vi "LabVIEW-Python-Interface_Example.vi"() -> ()   [LabVIEW 2016]
uses:
  pylvi/Controls/ArgumentType.ctl
  pylvi/Controls/DataType.ctl
  pylvi/Controls/ArgumentStructure.ctl
  pylvi/Controls/DescriptorStructure.ctl
  pylvi/PyLVi.lvclass
  <vilib>/Analysis/baseanly.llb/Mean (DBL).vi
  pylvi/argument_add/addArgument_Bool.vi
  pylvi/return_get/getReturn_Bool.vi
  pylvi/argument_add/addArgument_String.vi
  pylvi/return_get/getReturn_String.vi
  pylvi/argument_add/addArgument_Number_Float64.vi
  pylvi/return_get/getReturn_Number_Float64.vi
  pylvi/argument_add/addArgument_Number_Int32.vi
  pylvi/return_get/getReturn_Number_Int32.vi
  pylvi/argument_add/addArgument_Number_Complex128.vi
  pylvi/return_get/getReturn_Number_Complex128.vi
  pylvi/argument_add/addArgument_NumpyArray_Int32.vi
  pylvi/return_get/getReturn_NumpyArray_Int32.vi
  pylvi/argument_add/addArgument_NumpyArray_Float64.vi
  pylvi/return_get/getReturn_NumpyArray_Float64.vi
  pylvi/argument_add/addArgument_NumpyArray_Complex128.vi
  pylvi/return_get/getReturn_NumpyArray_Complex128.vi
  pylvi/argument_add/addArgument_NumpyArray2d_Int32.vi
  pylvi/return_get/getReturn_NumpyArray2d_Int32.vi
  pylvi/argument_add/addArgument_NumpyArray2d_Float64.vi
  pylvi/return_get/getReturn_NumpyArray2d_Float64.vi
  pylvi/argument_add/addArgument_NumpyArray2d_Complex128.vi
  pylvi/return_get/getReturn_NumpyArray2d_Complex128.vi
  pylvi/argument_add/addArgument_Dict.vi
  pylvi/return_get/getReturn_Dict.vi
  pylvi/attribute_set/setAttribute_Bool.vi
  pylvi/attribute_set/setAttribute_String.vi
  pylvi/attribute_set/setAttribute_Number_Int32.vi
  pylvi/attribute_set/setAttribute_Number_Float64.vi
  pylvi/attribute_set/setAttribute_Number_Complex128.vi
  pylvi/attribute_set/setAttribute_NumpyArray_Int32.vi
  pylvi/attribute_set/setAttribute_NumpyArray_Float64.vi
  pylvi/attribute_set/setAttribute_NumpyArray_Complex128.vi
  pylvi/attribute_set/setAttribute_NumpyArray2d_Int32.vi
  pylvi/attribute_set/setAttribute_NumpyArray2d_Float64.vi
  pylvi/attribute_set/setAttribute_NumpyArray2d_Complex128.vi
  pylvi/attribute_set/setAttribute_Dict.vi
  pylvi/attribute_get/getAttribute_Bool.vi
  pylvi/attribute_get/getAttribute_String.vi
  pylvi/attribute_get/getAttribute_Number_Int32.vi
  pylvi/attribute_get/getAttribute_Number_Float64.vi
  pylvi/attribute_get/getAttribute_Number_Complex128.vi
  pylvi/attribute_get/getAttribute_NumpyArray_Int32.vi
  pylvi/attribute_get/getAttribute_NumpyArray_Float64.vi
  pylvi/attribute_get/getAttribute_NumpyArray_Complex128.vi
  pylvi/attribute_get/getAttribute_NumpyArray2d_Int32.vi
  pylvi/attribute_get/getAttribute_NumpyArray2d_Float64.vi
  pylvi/attribute_get/getAttribute_NumpyArray2d_Complex128.vi
  pylvi/attribute_get/getAttribute_Dict.vi
  <vilib>/Analysis/NI_AALBase.lvlib
panel:
  in  "Tab Control":T1(tab)=enum."Single Argument Function Call"
  in  "open connection":bool
  in  "TCP address":string="tcp://127.0.0.1:5555"
  out "connection status":bool=TRUE
  in  "close connection":bool
  out "single:2darray receive complex":cdb[][](array[numeric])=[[2.0+0.0i, 2.0+0.0i, 4.0+0.0i, 4.0+0.0i]] caption="2darray receive complex"
  in  "single:2darray send complex":cdb[][](array[numeric])=[[2.17+0.25i, 2.0+0.0i, 4.0+0.88i, 4.0+0.0i], [0.5+0.0i, 85.6+0.0i, 7.2+1.52i, 0.0+0.0i]] caption="2darray send complex"
  out "single:array receive complex":cdb[](array[numeric]) caption="array receive complex"
  in  "single:array send complex":cdb[](array[numeric])=array[100005 elements] caption="array send complex"
  out "single:numeric receive complex":cdb caption="numeric receive complex"
  in  "single:numeric send complex":cdb=14.2+0.25i caption="numeric send complex"
  out "single:2darray receive":dbl[][](array[numeric])=[[2.0, 2.0, 4.0, 4.0]] caption="2darray receive"
  in  "single:2darray send":dbl[][](array[numeric])=[[0.85, 2.0, 4.0, 4.0], [0.0, 98.6, 9.58, 0.0]] caption="2darray send"
  in  "single:dict send":T2={"Name"="tcp://127.0.0.1:5555", "Number"=0.0, "Boolean"=FALSE, "Array"=[2.9, 2.0, 85.7, 4.01]} caption="dict send"
  out "single:dict receive":T2={"Name"="tcp://127.0.0.1:5555", "Number"=0.0, "Boolean"=FALSE, "Array"=[2.0, 2.0, 4.0, 4.0]} caption="dict receive"
  in  "single:function":string="fct_boolean" caption="function"
  in  "single:object":string="test" caption="object"
  in  "single:interations":i32=10 caption="interations"
  out "single:current iteration":i32=9 caption="current iteration"
  out "single:avg runtime [ms]":dbl=52.0 caption="avg runtime [ms]" format="%0.2f"
  in  "single argument fct call":bool
  in  "single:argtype":T3 caption="argtype"
  in  "single:data type":T4 caption="data type"
  in  "single:array send":dbl[](array[numeric])=[2.0, 2.99, 4.0, 4.869] caption="array send"
  out "single:array receive":dbl[](array[numeric]) caption="array receive"
  in  "single:bool send":bool caption="bool send"
  out "single:bool receive":bool caption="bool receive"
  in  "single:numeric send":dbl caption="numeric send"
  out "single:numeric receive":dbl caption="numeric receive"
  in  "single:string send":string caption="string send"
  out "single:string receive":string caption="string receive"
  out "multi:2darray receive complex":cdb[][](array[numeric])=[[4.0+170.6i, 4.0+0.2i, 8.0+1.6i, 8.0+0.0i], [0.0+0.0i, 3.0+104.0i, 0.0+1.1i, 0.0+0.0i]] caption="2darray receive complex"
  in  "multi:2darray send complex":cdb[][](array[numeric])=[[2.0+85.3i, 2.0+0.1i, 4.0+0.8i, 4.0+0.0i], [0.0+0.0i, 1.5+52.0i, 0.0+0.55i, 0.0+0.0i]] caption="2darray send complex"
  out "multi:array receive complex":cdb[](array[numeric])=[4.34+0.0i, 4.0+0.0i, 8.0+1.16i, 8.6+0.2i] caption="array receive complex"
  in  "multi:array send complex":cdb[](array[numeric])=[2.17+0.0i, 2.0+0.0i, 4.0+0.58i, 4.3+0.1i] caption="array send complex"
  out "multi:numeric receive complex":cdb=0.4+11.6i caption="numeric receive complex"
  in  "multi:numeric send complex":cdb=0.2+5.8i caption="numeric send complex"
  in  "multi:clear last argument":bool
  out "multi:argument receive":T5[](array[typedef])
  out "multi:2darray receive":dbl[][](array[numeric]) caption="2darray receive"
  out "multi:dict receive":T2={"Name"="tcp://127.0.0.1:5555", "Number"=0.0, "Boolean"=FALSE, "Array"=[2.0, 2.0, 4.0, 4.0]} caption="dict receive"
  out "multi:array receive":dbl[](array[numeric]) caption="array receive"
  out "multi:bool receive":bool caption="bool receive"
  out "multi:numeric receive":dbl caption="numeric receive"
  out "multi:string receive":string caption="string receive"
  in  "multi:get return parameter":bool
  in  "multi:add argument":bool
  in  "multi:call function":bool
  in  "multi:2darray send":dbl[][](array[numeric])=[[2.17, 2.0, 4.9, 4.0], [0.0, 8.5, 0.0, 0.0]] caption="2darray send"
  in  "multi:dict send":T2={"Name"="tcp://127.0.0.1:5555", "Number"=0.0, "Boolean"=FALSE, "Array"=[2.0, 2.0, 4.0, 4.0]} caption="dict send"
  in  "multi:array send":dbl[](array[numeric])=[28.5, 2.0, 85.3, 4.0] caption="array send"
  in  "multi:bool send":bool caption="bool send"
  in  "multi:numeric send":dbl caption="numeric send"
  in  "multi:string send":string caption="string send"
  in  "multi:function":string="multi_array_test" caption="function"
  in  "multi:object":string="test" caption="object"
  in  "multi:argtype":T3 caption="argtype"
  in  "multi:data type":T4 caption="data type"
  out "multi:argument send":T5[](array[typedef])
  out "prop:2darray receive complex":cdb[][](array[numeric])=[[2.0+0.0i, 2.0+0.0i, 4.0+0.0i, 4.0+0.0i], [0.0+0.0i, 0.0+0.0i, 1.2+0.22i, 0.0+0.0i]] caption="2darray get complex"
  in  "prop:2darray set complex":cdb[][](array[numeric])=[[2.0+0.25i, 2.68+17.2i, 4.0+0.98i, 4.0+0.0i], [8.6+52.8i, 0.0+0.0i, 1.2+0.22i, 0.0+0.0i]] caption="2darray set complex"
  out "prop:array get complex":cdb[](array[numeric])=[2.1+0.0i, 2.0+0.1i, 4.0+0.2i, 4.0+17.2i] caption="array get complex"
  in  "prop:array set complex":cdb[](array[numeric])=[2.1+0.0i, 2.0+0.1i, 4.0+0.2i, 4.0+17.2i] caption="array set complex"
  out "prop:numeric get complex":cdb=7.2+17.23i caption="numeric get complex"
  in  "prop:numeric set complex":cdb=25.5+0.72i caption="numeric set complex"
  out "prop:2darray get":dbl[][](array[numeric])=[[2.0, 2.0, 4.0, 4.0]] caption="2darray get"
  out "prop:dict get":T2={"Name"="tcp://127.0.0.1:5555", "Number"=0.0, "Boolean"=FALSE, "Array"=[2.0, 2.0, 4.0, 4.0]} caption="dict get"
  out "prop:array get":dbl[](array[numeric]) caption="array get"
  out "prop:bool get":bool caption="bool get"
  out "prop:numeric get":dbl caption="numeric get"
  out "grop:string get":string caption="string get"
  in  "prop:get":bool
  in  "prop:set":bool
  in  "prop:2darray set":dbl[][](array[numeric])=[[2.17, 2.9, 4.0, 4.0], [0.33, 0.0, 17.5, 0.0]] caption="2darray set"
  in  "prop:array set":dbl[](array[numeric])=[2.0, 2.0, 4.0, 4.0] caption="array set"
  in  "prop:dict set":T2={"Name"="tcp://127.0.0.1:5555", "Number"=0.0, "Boolean"=FALSE, "Array"=[2.5, 18.5, 8.5, 4.0]} caption="dict set"
  in  "prop:bool set":bool caption="bool set"
  in  "prop:numeric set":dbl caption="numeric set"
  in  "prop:string set":string caption="string set"
  in  "prop:property":string="var_double" caption="property/attribute"
  in  "prop:object":string="test" caption="object"
  in  "prop:argtype":T3=enum."numeric" caption="argtype"
  in  "prop:data type":T4=enum."float64" caption="data type"
  in  "stop":bool
  # "A function with a single parameter is called. This function returns the same value or a modified one."
  # "Benchmarking"
  # "1. Add arguments\n2. Call function\n3. Parse return parameters"
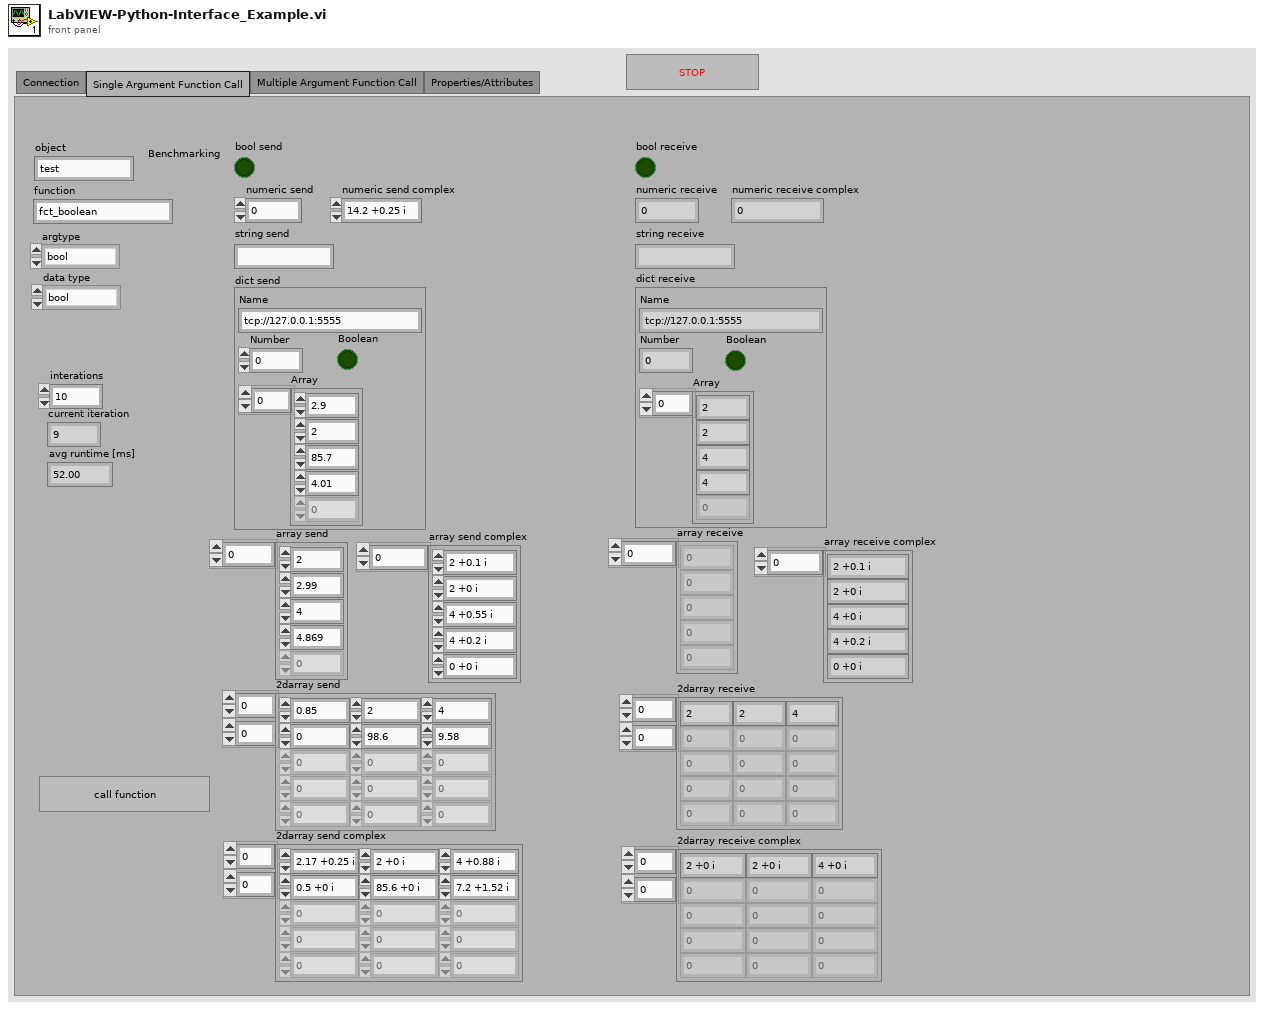
[diagram p1: front panel]
types:
  T1 = enum32{"Connection", "Single Argument Function Call", "Multiple Argument Function Call", "Properties/Attributes"}
  T2 = cluster{"Name":string, "Number":dbl, "Boolean":bool, "Array":dbl[]}
  T3 = typedef "PyLVi.lvlib/PyLVi.lvclass/ArgumentType.ctl" = enum8{"bool", "numeric", "string", "dict", "ndarray", "ndarray2d"}
  T4 = typedef "PyLVi.lvlib/PyLVi.lvclass/DataType.ctl" = enum16{"bool", "string", "int16", "int32", "float32", "float64", "complex128"}
  T5 = typedef "PyLVi.lvlib/PyLVi.lvclass/ArgumentStructure.ctl" = cluster{"descriptor structure":T6, "data string":string}
  T6 = typedef "PyLVi.lvlib/PyLVi.lvclass/DescriptorStructure.ctl" = cluster{"argtype":string, "dtype":string, "shape":u32[], "argname":string}
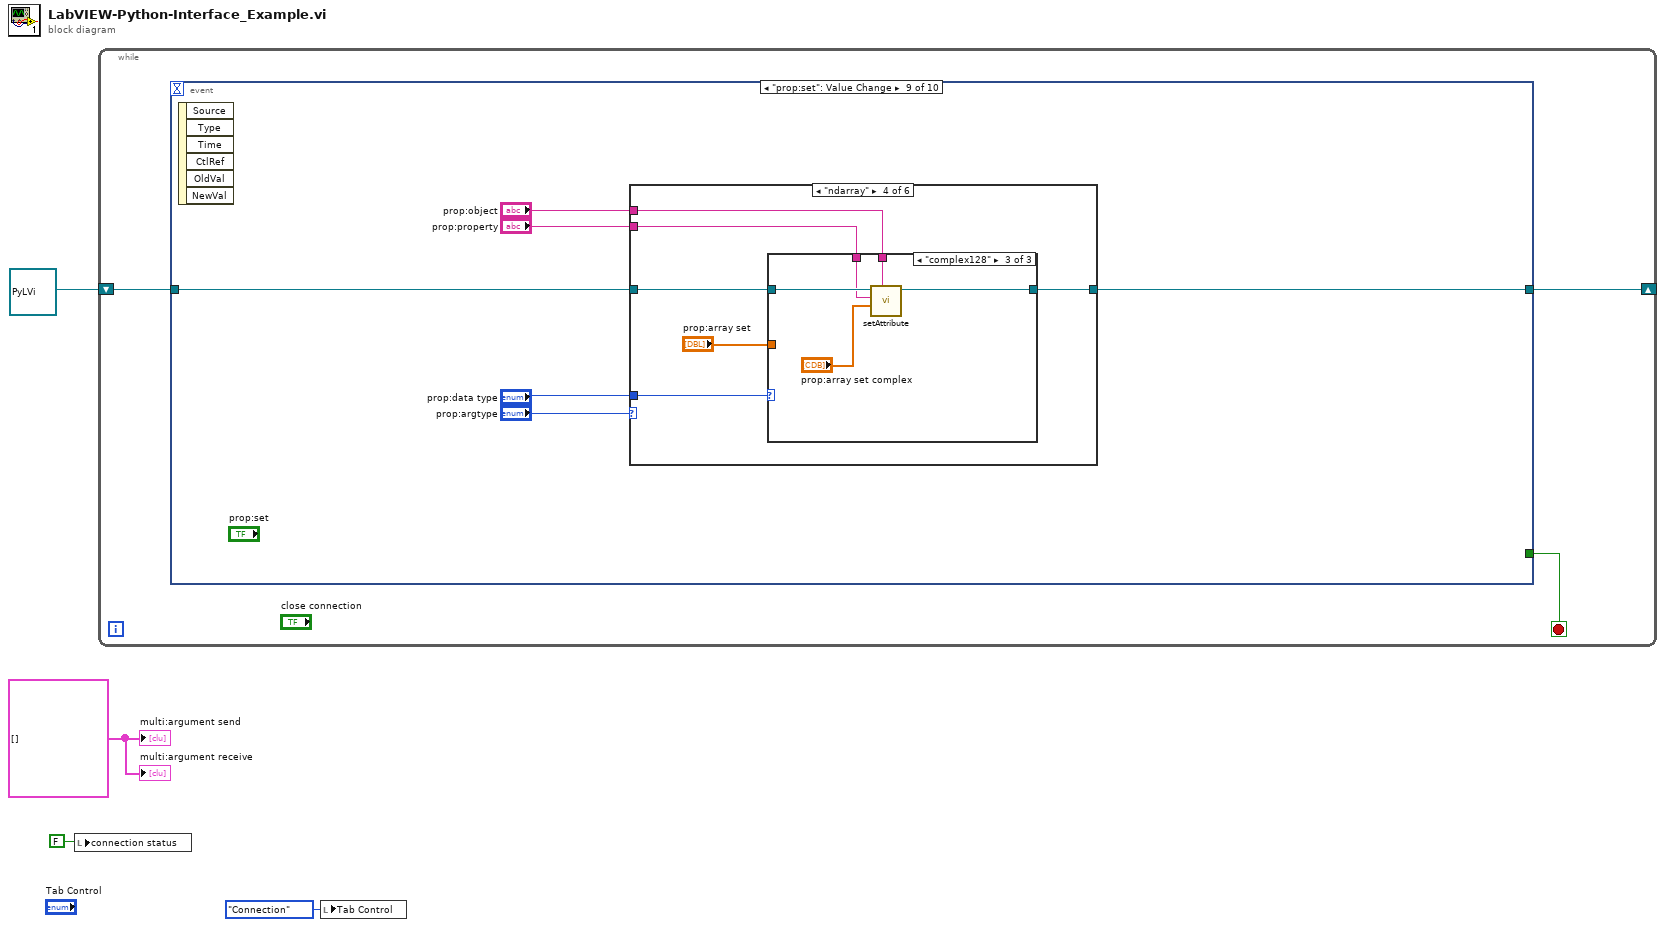
[diagram p0: block diagram]
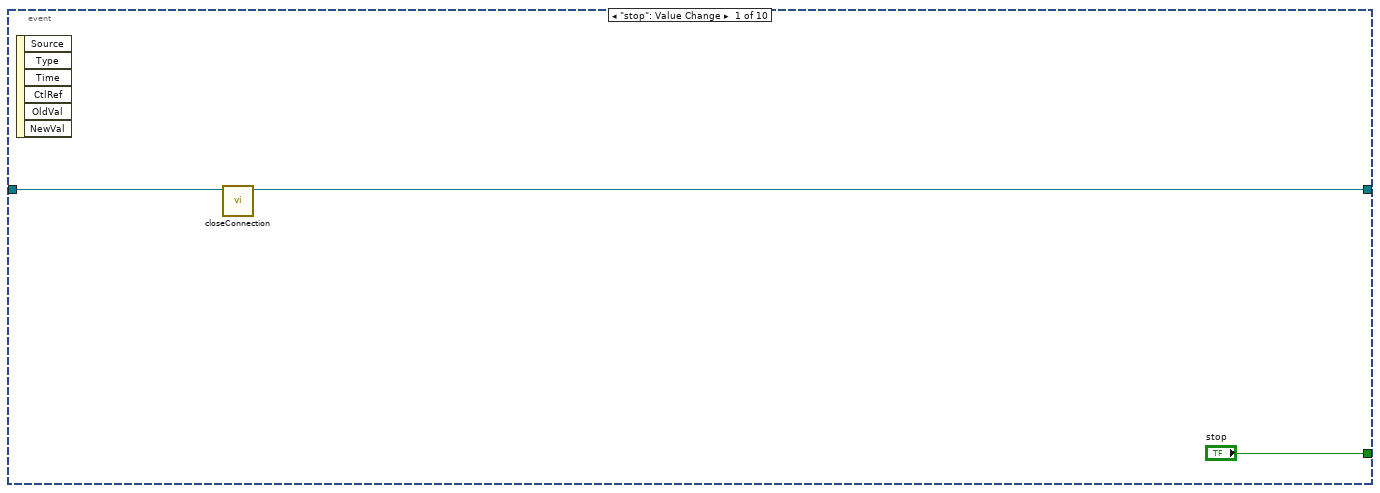
[diagram p2: hidden frame]
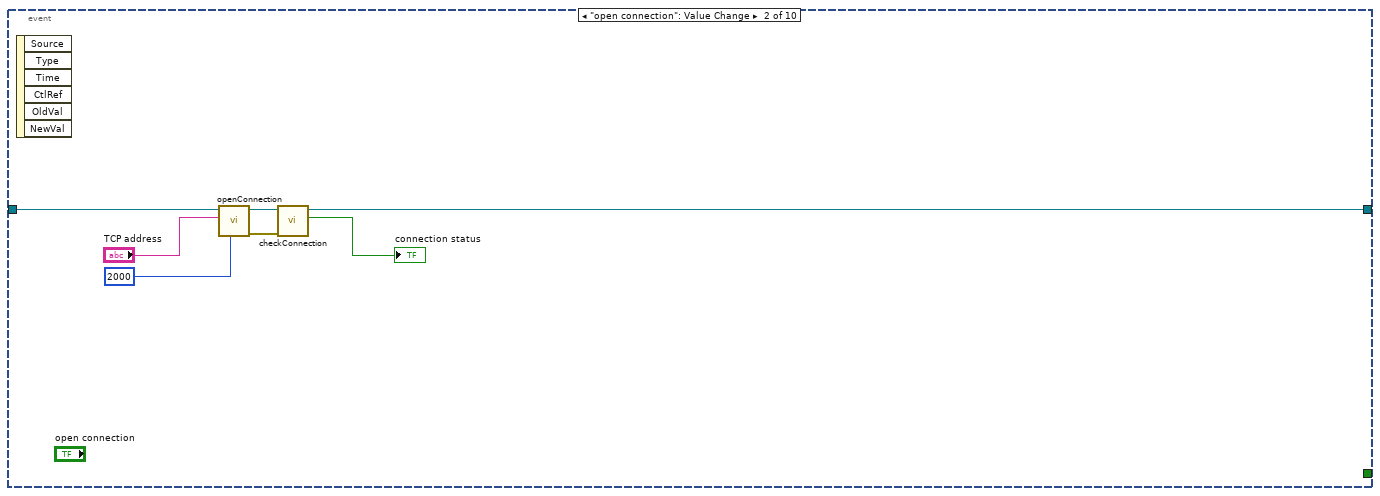
[diagram p3: hidden frame]
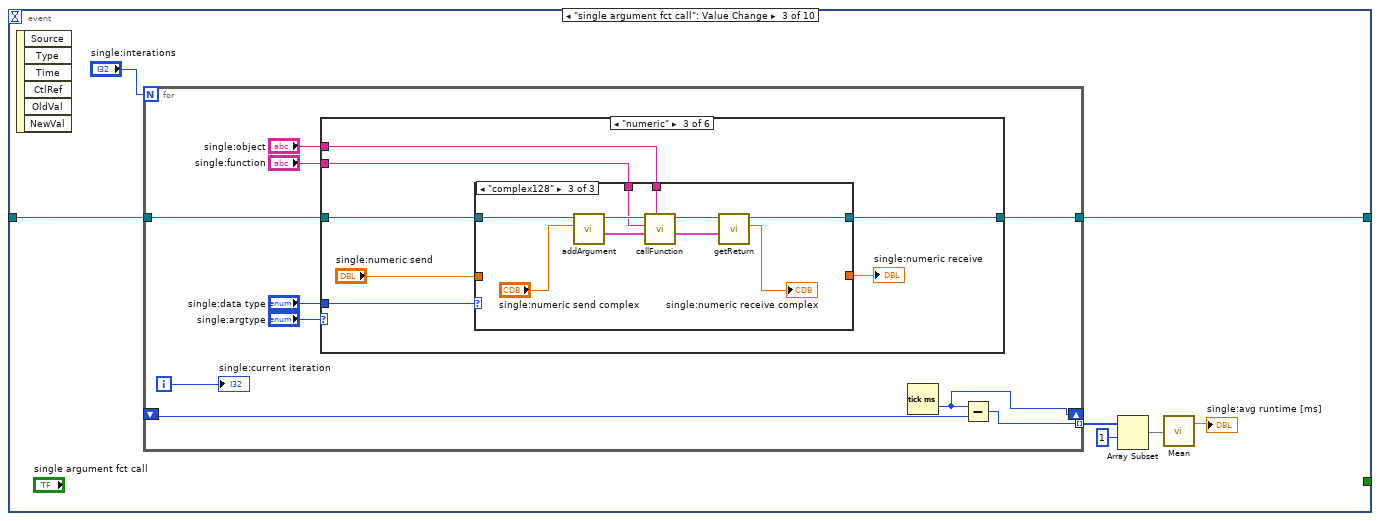
[diagram p4: hidden frame]
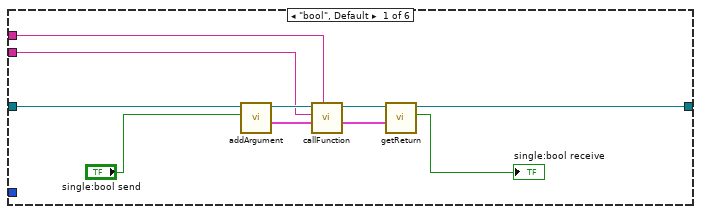
[diagram p5: hidden frame]
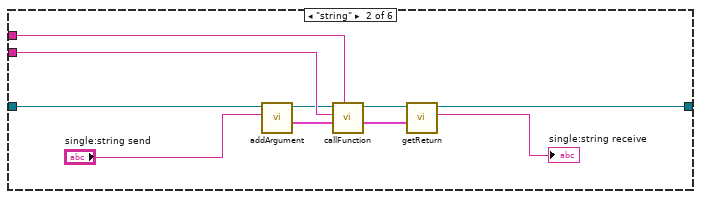
[diagram p6: hidden frame]
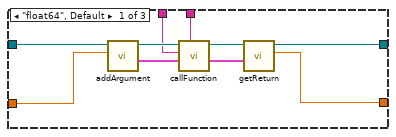
[diagram p7: hidden frame]
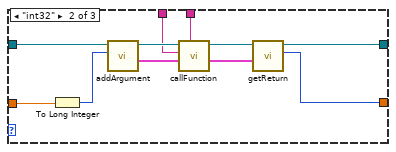
[diagram p8: hidden frame]
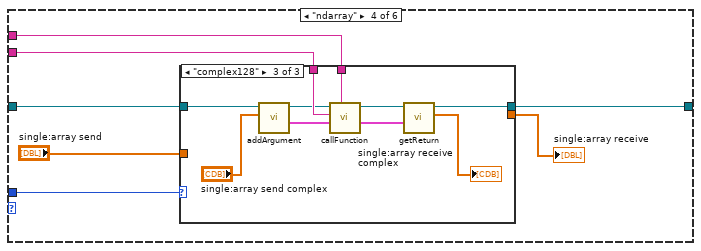
[diagram p9: hidden frame]
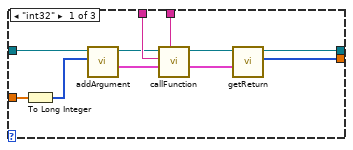
[diagram p10: hidden frame]
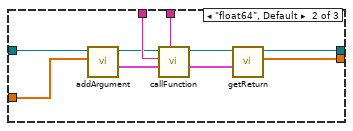
[diagram p11: hidden frame]
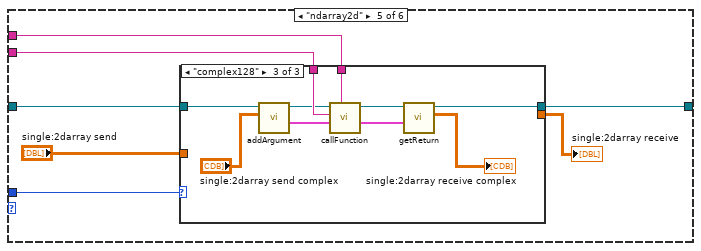
[diagram p12: hidden frame]
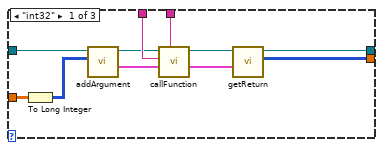
[diagram p13: hidden frame]
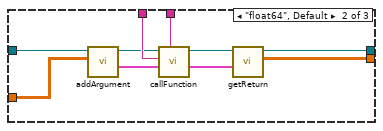
[diagram p14: hidden frame]
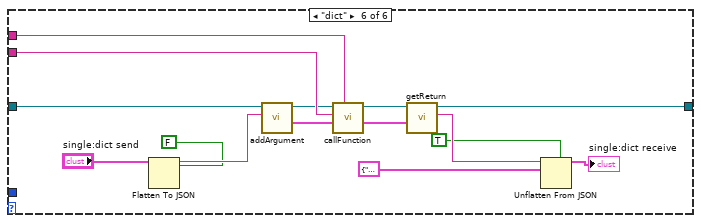
[diagram p15: hidden frame]
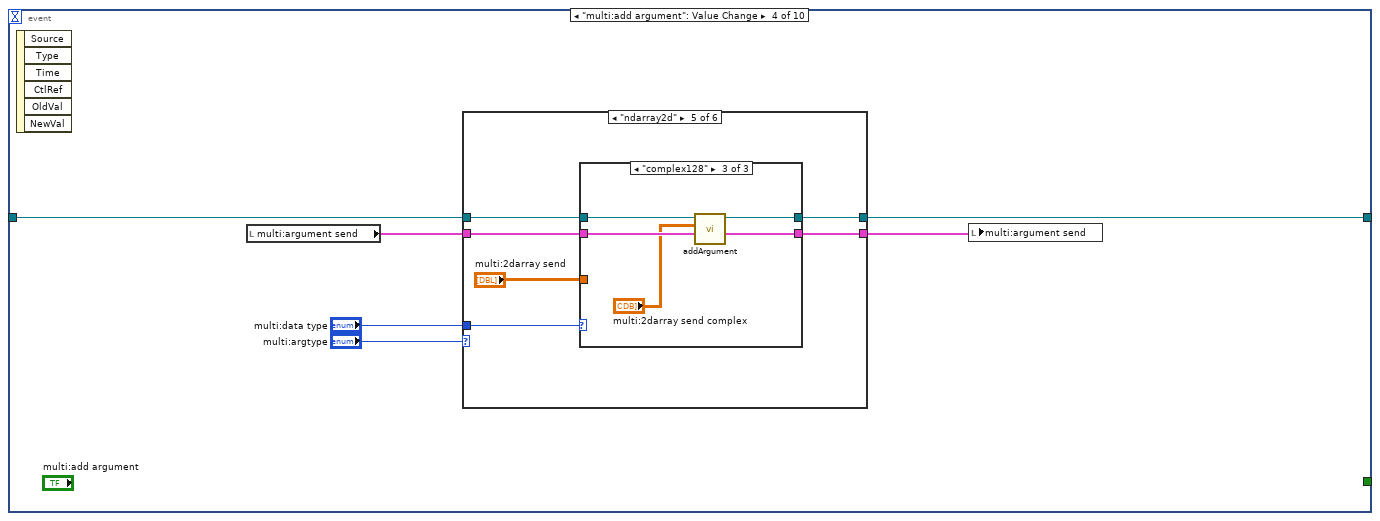
[diagram p16: hidden frame]
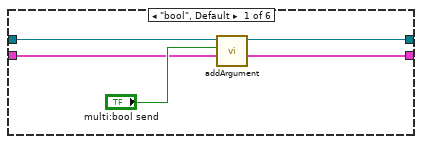
[diagram p17: hidden frame]
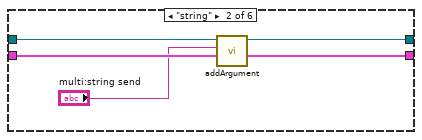
[diagram p18: hidden frame]
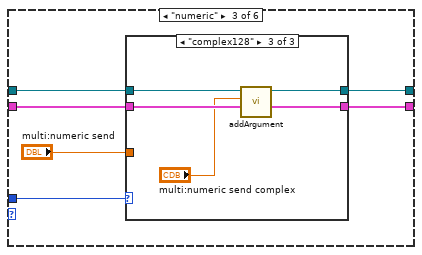
[diagram p19: hidden frame]
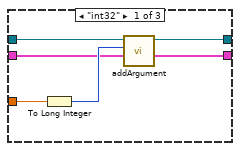
[diagram p20: hidden frame]
diagram:
  w2 = T5[] [] ("multi:argument send")
  n1 = local write "connection status"(FALSE ("status")) -> ()
  n2 = while {
    shift-right: [w6] -> _
    shift-left: refnum<class "PyLVi.lvclass"> refnum ("Python_LabView_Interface:Python-Labview_Communication.lvclass") -> [w5]
    stop <- w7 stop-if-true
    n3 = event shown="[8] \"prop:set\": Value Change" {
      selector: _ -> [_ _ _ _ _ _ _ _ _ _]
      dyn-events: _ -> [_ _ _ _ _ _ _ _ _ _]
      timeout: _ -> [_ _ _ _ _ _ _ _ _ _]
      tunnel: ["stop" _ _ _ _ _ _ _ _ _] -> w7
      tunnel: w5 -> [w9 w17 w24 w189 w273 w284 w290 w373 w378 w468]
      tunnel: [w8 w12 w23 w188 w273 w283 w289 w372 w374 w467] -> w6
      event "stop": Value Change {
        n4 = event-data() -> ()  [unwired: 1 in, 6 out]
        n5 = call "closeConnection.vi"("LabVIEW-Python-Interface in"=w9) -> ("LabVIEW-Python-Interface out"=w8:refnum<class "PyLVi.lvclass">)  [unwired: 9 in, 1 out]
      }
      event "open connection": Value Change {
        n6 = event-data() -> ()  [unwired: 1 in, 6 out]
        n7 = call "openConnection.vi"("recveive timeout"=2000, "TCP address"="TCP address", "LabVIEW-Python-Interface in"=w17) -> ("error out"=w14:errorcluster, "LabVIEW-Python-Interface out"=w15:refnum<class "PyLVi.lvclass">)  [unwired: 6 in, 1 out]
        n8 = call "checkConnection.vi"("error in (no error)"=w14, "LabVIEW-Python-Interface in"=w15) -> ("connection established"=→"connection status":bool, "LabVIEW-Python-Interface out"=w12:refnum<class "PyLVi.lvclass">)  [unwired: 7 in, 1 out]
      }
      event "single argument fct call": Value Change {
        n9 = event-data() -> ()  [unwired: 1 in, 6 out]
        n10 = for {
          N: "single:interations" -> [_]
          tunnel: w24 -> [w30]
          tunnel: [w31] -> w23
          shift-right: [w33] -> _
          shift-left: _ -> [w34]
          tunnel: [w32] -> w20 mode=indexing
          i -> [w25]
          n11 = case shown="\"numeric\"" "single:argtype" {
            tunnel: [w39 w53 w60 w99 w137 w182] -> w31
            tunnel: w30 -> [w40 w54 w61 w98 w136 w183]
            tunnel: "single:object" -> [w38 w52 w59 w97 w135 w181]
            tunnel: "single:function" -> [w37 w51 w58 w96 w134 w180]
            tunnel: "single:data type" -> [_ _ w57 w95 w133 _]
            frame "bool", Default {
              n12 = call-poly "addArgument.vi"("data"="single:bool send", "LabVIEW-Python-Interface in"=w40) -> ("argument list out"=w43:T5[], "LabVIEW-Python-Interface out"=w44:refnum<class "PyLVi.lvclass">)  [unwired: 7 in, 1 out]
              n13 = call "callFunction.vi"("object"=w38, "argument list in"=w43, "function"=w37, "LabVIEW-Python-Interface in"=w44) -> ("return list"=w41:T5[], "LabVIEW-Python-Interface out"=w42:refnum<class "PyLVi.lvclass">)  [unwired: 5 in, 1 out]
              n14 = call-poly "getReturn.vi"("return list in"=w41, "LabVIEW-Python-Interface in"=w42) -> ("data"=→"single:bool receive":bool, "LabVIEW-Python-Interface out"=w39:refnum<class "PyLVi.lvclass">)  [unwired: 6 in, 2 out]
            }
            frame "string" {
              n15 = call-poly "addArgument.vi"("data"="single:string send", "LabVIEW-Python-Interface in"=w54) -> ("argument list out"=w49:T5[], "LabVIEW-Python-Interface out"=w50:refnum<class "PyLVi.lvclass">)  [unwired: 7 in, 1 out]
              n16 = call "callFunction.vi"("object"=w52, "argument list in"=w49, "function"=w51, "LabVIEW-Python-Interface in"=w50) -> ("return list"=w47:T5[], "LabVIEW-Python-Interface out"=w48:refnum<class "PyLVi.lvclass">)  [unwired: 5 in, 1 out]
              n17 = call-poly "getReturn.vi"("return list in"=w47, "LabVIEW-Python-Interface in"=w48) -> ("data out"=→"single:string receive":string, "LabVIEW-Python-Interface out"=w53:refnum<class "PyLVi.lvclass">)  [unwired: 6 in, 2 out]
            }
            frame "numeric" {
              n18 = case shown="\"complex128\"" w57 {
                tunnel: w61 -> [w67 w78 w88]
                tunnel: [w66 w77 w87] -> w60
                tunnel: w59 -> [w65 w76 w86]
                tunnel: w58 -> [w64 w75 w85]
                tunnel: "single:numeric send" -> [w62 w72 _]
                tunnel: [w63 w74 _] -> w55
                frame "float64", Default {
                  n19 = call-poly "addArgument.vi"("data"=w62, "LabVIEW-Python-Interface in"=w67) -> ("argument list out"=w70:T5[], "LabVIEW-Python-Interface out"=w71:refnum<class "PyLVi.lvclass">)  [unwired: 7 in, 1 out]
                  n20 = call "callFunction.vi"("object"=w65, "argument list in"=w70, "function"=w64, "LabVIEW-Python-Interface in"=w71) -> ("return list"=w68:T5[], "LabVIEW-Python-Interface out"=w69:refnum<class "PyLVi.lvclass">)  [unwired: 5 in, 1 out]
                  n21 = call-poly "getReturn.vi"("return list in"=w68, "LabVIEW-Python-Interface in"=w69) -> ("data out"=w63:dbl, "LabVIEW-Python-Interface out"=w66:refnum<class "PyLVi.lvclass">)  [unwired: 6 in, 2 out]
                }
                frame "int32" {
                  n22 = To Long Integer(number=w72) -> (32bit integer=w73:i32)
                  n23 = call-poly "addArgument.vi"("data"=w73, "LabVIEW-Python-Interface in"=w78) -> ("argument list out"=w81:T5[], "LabVIEW-Python-Interface out"=w82:refnum<class "PyLVi.lvclass">)  [unwired: 7 in, 1 out]
                  n24 = call "callFunction.vi"("object"=w76, "argument list in"=w81, "function"=w75, "LabVIEW-Python-Interface in"=w82) -> ("return list"=w79:T5[], "LabVIEW-Python-Interface out"=w80:refnum<class "PyLVi.lvclass">)  [unwired: 5 in, 1 out]
                  n25 = call-poly "getReturn.vi"("return list in"=w79, "LabVIEW-Python-Interface in"=w80) -> ("data out"=w74:i32, "LabVIEW-Python-Interface out"=w77:refnum<class "PyLVi.lvclass">)  [unwired: 6 in, 2 out]
                }
                frame "complex128" {
                  n26 = call-poly "addArgument.vi"("data"="single:numeric send complex", "LabVIEW-Python-Interface in"=w88) -> ("argument list out"=w91:T5[], "LabVIEW-Python-Interface out"=w92:refnum<class "PyLVi.lvclass">)  [unwired: 7 in, 1 out]
                  n27 = call "callFunction.vi"("object"=w86, "argument list in"=w91, "function"=w85, "LabVIEW-Python-Interface in"=w92) -> ("return list"=w89:T5[], "LabVIEW-Python-Interface out"=w90:refnum<class "PyLVi.lvclass">)  [unwired: 5 in, 1 out]
                  n28 = call-poly "getReturn.vi"("return list in"=w89, "LabVIEW-Python-Interface in"=w90) -> ("data out"=→"single:numeric receive complex":cdb, "LabVIEW-Python-Interface out"=w87:refnum<class "PyLVi.lvclass">)  [unwired: 6 in, 2 out]
                }
              }
              "single:numeric receive" <- w55
            }
            frame "ndarray" {
              n29 = case shown="\"complex128\"" w95 {
                tunnel: [w102 w114 w124] -> w99
                tunnel: w98 -> [w107 w118 w128]
                tunnel: w97 -> [w110 w120 w130]
                tunnel: w96 -> [w109 w119 w129]
                tunnel: "single:array send" -> [w108 w111 _]
                tunnel: [w100 w112 _] -> w93
                frame "int32" {
                  n30 = To Long Integer(number=w108) -> (32bit integer=w104:i32[])
                  n31 = call-poly "addArgument.vi"("data"=w104, "LabVIEW-Python-Interface in"=w107) -> ("argument list out"=w105:T5[], "LabVIEW-Python-Interface out"=w106:refnum<class "PyLVi.lvclass">)  [unwired: 7 in, 1 out]
                  n32 = call "callFunction.vi"("object"=w110, "argument list in"=w105, "function"=w109, "LabVIEW-Python-Interface in"=w106) -> ("return list"=w101:T5[], "LabVIEW-Python-Interface out"=w103:refnum<class "PyLVi.lvclass">)  [unwired: 5 in, 1 out]
                  n33 = call-poly "getReturn.vi"("return list in"=w101, "LabVIEW-Python-Interface in"=w103) -> ("data out"=w100:i32[], "LabVIEW-Python-Interface out"=w102:refnum<class "PyLVi.lvclass">)  [unwired: 6 in, 2 out]
                }
                frame "float64", Default {
                  n34 = call-poly "addArgument.vi"("data"=w111, "LabVIEW-Python-Interface in"=w118) -> ("argument list out"=w116:T5[], "LabVIEW-Python-Interface out"=w117:refnum<class "PyLVi.lvclass">)  [unwired: 7 in, 1 out]
                  n35 = call "callFunction.vi"("object"=w120, "argument list in"=w116, "function"=w119, "LabVIEW-Python-Interface in"=w117) -> ("return list"=w113:T5[], "LabVIEW-Python-Interface out"=w115:refnum<class "PyLVi.lvclass">)  [unwired: 5 in, 1 out]
                  n36 = call-poly "getReturn.vi"("return list in"=w113, "LabVIEW-Python-Interface in"=w115) -> ("data out"=w112:dbl[], "LabVIEW-Python-Interface out"=w114:refnum<class "PyLVi.lvclass">)  [unwired: 6 in, 2 out]
                }
                frame "complex128" {
                  n37 = call-poly "addArgument.vi"("data"="single:array send complex", "LabVIEW-Python-Interface in"=w128) -> ("argument list out"=w126:T5[], "LabVIEW-Python-Interface out"=w127:refnum<class "PyLVi.lvclass">)  [unwired: 7 in, 1 out]
                  n38 = call "callFunction.vi"("object"=w130, "argument list in"=w126, "function"=w129, "LabVIEW-Python-Interface in"=w127) -> ("return list"=w123:T5[], "LabVIEW-Python-Interface out"=w125:refnum<class "PyLVi.lvclass">)  [unwired: 5 in, 1 out]
                  n39 = call-poly "getReturn.vi"("return list in"=w123, "LabVIEW-Python-Interface in"=w125) -> ("data out"=→"single:array receive complex":cdb[], "LabVIEW-Python-Interface out"=w124:refnum<class "PyLVi.lvclass">)  [unwired: 6 in, 2 out]
                }
              }
              "single:array receive" <- w93
            }
            frame "ndarray2d" {
              n40 = case shown="\"complex128\"" w133 {
                tunnel: [w140 w152 w162] -> w137
                tunnel: w136 -> [w145 w156 w166]
                tunnel: w135 -> [w148 w158 w168]
                tunnel: w134 -> [w147 w157 w167]
                tunnel: "single:2darray send" -> [w146 w149 _]
                tunnel: [w138 w150 _] -> w131
                frame "int32" {
                  n41 = To Long Integer(number=w146) -> (32bit integer=w142:i32[][])
                  n42 = call-poly "addArgument.vi"("data"=w142, "LabVIEW-Python-Interface in"=w145) -> ("argument list out"=w143:T5[], "LabVIEW-Python-Interface out"=w144:refnum<class "PyLVi.lvclass">)  [unwired: 7 in, 1 out]
                  n43 = call "callFunction.vi"("object"=w148, "argument list in"=w143, "function"=w147, "LabVIEW-Python-Interface in"=w144) -> ("return list"=w139:T5[], "LabVIEW-Python-Interface out"=w141:refnum<class "PyLVi.lvclass">)  [unwired: 5 in, 1 out]
                  n44 = call-poly "getReturn.vi"("return list in"=w139, "LabVIEW-Python-Interface in"=w141) -> ("data out"=w138:i32[][], "LabVIEW-Python-Interface out"=w140:refnum<class "PyLVi.lvclass">)  [unwired: 6 in, 2 out]
                }
                frame "float64", Default {
                  n45 = call-poly "addArgument.vi"("data"=w149, "LabVIEW-Python-Interface in"=w156) -> ("argument list out"=w154:T5[], "LabVIEW-Python-Interface out"=w155:refnum<class "PyLVi.lvclass">)  [unwired: 7 in, 1 out]
                  n46 = call "callFunction.vi"("object"=w158, "argument list in"=w154, "function"=w157, "LabVIEW-Python-Interface in"=w155) -> ("return list"=w151:T5[], "LabVIEW-Python-Interface out"=w153:refnum<class "PyLVi.lvclass">)  [unwired: 5 in, 1 out]
                  n47 = call-poly "getReturn.vi"("return list in"=w151, "LabVIEW-Python-Interface in"=w153) -> ("data out"=w150:dbl[][], "LabVIEW-Python-Interface out"=w152:refnum<class "PyLVi.lvclass">)  [unwired: 6 in, 2 out]
                }
                frame "complex128" {
                  n48 = call-poly "addArgument.vi"("data"="single:2darray send complex", "LabVIEW-Python-Interface in"=w166) -> ("argument list out"=w164:T5[], "LabVIEW-Python-Interface out"=w165:refnum<class "PyLVi.lvclass">)  [unwired: 7 in, 1 out]
                  n49 = call "callFunction.vi"("object"=w168, "argument list in"=w164, "function"=w167, "LabVIEW-Python-Interface in"=w165) -> ("return list"=w161:T5[], "LabVIEW-Python-Interface out"=w163:refnum<class "PyLVi.lvclass">)  [unwired: 5 in, 1 out]
                  n50 = call-poly "getReturn.vi"("return list in"=w161, "LabVIEW-Python-Interface in"=w163) -> ("data out"=→"single:2darray receive complex":cdb[][], "LabVIEW-Python-Interface out"=w162:refnum<class "PyLVi.lvclass">)  [unwired: 6 in, 2 out]
                }
              }
              "single:2darray receive" <- w131
            }
            frame "dict" {
              n51 = Flatten To JSON(enable LabVIEW extensions? (T)=FALSE, anything="single:dict send") -> (JSON string=w174:string)  [unwired: 1 in, 1 out]
              n52 = call-poly "addArgument.vi"("JSON string"=w174, "LabVIEW-Python-Interface in"=w183) -> ("argument list out"=w178:T5[], "LabVIEW-Python-Interface out"=w179:refnum<class "PyLVi.lvclass">)  [unwired: 7 in, 1 out]
              n53 = call "callFunction.vi"("object"=w181, "argument list in"=w178, "function"=w180, "LabVIEW-Python-Interface in"=w179) -> ("return list"=w176:T5[], "LabVIEW-Python-Interface out"=w177:refnum<class "PyLVi.lvclass">)  [unwired: 5 in, 1 out]
              n54 = call-poly "getReturn.vi"("return list in"=w176, "LabVIEW-Python-Interface in"=w177) -> ("data out"=w175:string, "LabVIEW-Python-Interface out"=w182:refnum<class "PyLVi.lvclass">)  [unwired: 6 in, 2 out]
              n55 = Unflatten From JSON(enable LabVIEW extensions? (T)=TRUE, JSON string=w175, type and defaults=T2 {"Name"="tcp://127.0.0.1:5555", "Number"=0.0, "Boolean"=FALSE, "Array"=[2.0, 2.0, 4.0, 4.0]} ("single:dict receive")) -> (value=→"single:dict receive":T2)  [unwired: 4 in, 1 out]
            }
          }
          n56 = Tick Count (ms)() -> (millisecond timer value=w33:u32)
          n57 = Subtract(x=w33, y=w34) -> (x-y=w32:u32)
          "single:current iteration" <- w25
        }
        n58 = Array Subset(array=w20, index=1) -> (w21:u32[])  [unwired: 1 in]
        n59 = call-poly <vilib>:"Mean.vi"("X"=w21) -> ("mean"=→"single:avg runtime [ms]":dbl)  [unwired: 1 out]
      }
      event "multi:add argument": Value Change {
        n60 = event-data() -> ()  [unwired: 1 in, 6 out]
        n61 = local read "multi:argument send"() -> (w184:T5[])
        n62 = case shown="\"ndarray2d\"" "multi:argtype" {
          tunnel: w189 -> [w194 w199 w205 w227 w249 w272]
          tunnel: [w193 w198 w204 w226 w248 w271] -> w188
          tunnel: "multi:data type" -> [_ _ w203 w225 w247 _]
          tunnel: [w191 w197 w202 w224 w246 w270] -> w185
          tunnel: w184 -> [w190 w196 w200 w223 w245 w269]
          frame "bool", Default {
            n63 = call-poly "addArgument.vi"("argument list in"=w190, "data"="multi:bool send", "LabVIEW-Python-Interface in"=w194) -> ("argument list out"=w191:T5[], "LabVIEW-Python-Interface out"=w193:refnum<class "PyLVi.lvclass">)  [unwired: 6 in, 1 out]
          }
          frame "string" {
            n64 = call-poly "addArgument.vi"("argument list in"=w196, "data"="multi:string send", "LabVIEW-Python-Interface in"=w199) -> ("argument list out"=w197:T5[], "LabVIEW-Python-Interface out"=w198:refnum<class "PyLVi.lvclass">)  [unwired: 6 in, 1 out]
          }
          frame "numeric" {
            n65 = case shown="\"complex128\"" w203 {
              tunnel: w205 -> [w211 w216 w221]
              tunnel: [w210 w215 w220] -> w204
              tunnel: [w209 w214 w219] -> w202
              tunnel: "multi:numeric send" -> [w208 w213 _]
              tunnel: w200 -> [w206 w212 w218]
              frame "int32" {
                n66 = To Long Integer(number=w208) -> (32bit integer=w207:i32)
                n67 = call-poly "addArgument.vi"("argument list in"=w206, "data"=w207, "LabVIEW-Python-Interface in"=w211) -> ("argument list out"=w209:T5[], "LabVIEW-Python-Interface out"=w210:refnum<class "PyLVi.lvclass">)  [unwired: 6 in, 1 out]
              }
              frame "float64", Default {
                n68 = call-poly "addArgument.vi"("argument list in"=w212, "data"=w213, "LabVIEW-Python-Interface in"=w216) -> ("argument list out"=w214:T5[], "LabVIEW-Python-Interface out"=w215:refnum<class "PyLVi.lvclass">)  [unwired: 6 in, 1 out]
              }
              frame "complex128" {
                n69 = call-poly "addArgument.vi"("argument list in"=w218, "data"="multi:numeric send complex", "LabVIEW-Python-Interface in"=w221) -> ("argument list out"=w219:T5[], "LabVIEW-Python-Interface out"=w220:refnum<class "PyLVi.lvclass">)  [unwired: 6 in, 1 out]
              }
            }
          }
          frame "ndarray" {
            n70 = case shown="\"complex128\"" w225 {
              tunnel: w227 -> [w233 w238 w243]
              tunnel: [w232 w237 w242] -> w226
              tunnel: [w231 w236 w241] -> w224
              tunnel: "multi:array send" -> [w230 w235 _]
              tunnel: w223 -> [w228 w234 w240]
              frame "int32" {
                n71 = To Long Integer(number=w230) -> (32bit integer=w229:i32[])
                n72 = call-poly "addArgument.vi"("argument list in"=w228, "data"=w229, "LabVIEW-Python-Interface in"=w233) -> ("argument list out"=w231:T5[], "LabVIEW-Python-Interface out"=w232:refnum<class "PyLVi.lvclass">)  [unwired: 6 in, 1 out]
              }
              frame "float64", Default {
                n73 = call-poly "addArgument.vi"("argument list in"=w234, "data"=w235, "LabVIEW-Python-Interface in"=w238) -> ("argument list out"=w236:T5[], "LabVIEW-Python-Interface out"=w237:refnum<class "PyLVi.lvclass">)  [unwired: 6 in, 1 out]
              }
              frame "complex128" {
                n74 = call-poly "addArgument.vi"("argument list in"=w240, "data"="multi:array send complex", "LabVIEW-Python-Interface in"=w243) -> ("argument list out"=w241:T5[], "LabVIEW-Python-Interface out"=w242:refnum<class "PyLVi.lvclass">)  [unwired: 6 in, 1 out]
              }
            }
          }
          frame "ndarray2d" {
            n75 = case shown="\"complex128\"" w247 {
              tunnel: w249 -> [w255 w260 w265]
              tunnel: [w254 w259 w264] -> w248
              tunnel: [w253 w258 w263] -> w246
              tunnel: "multi:2darray send" -> [w252 w257 _]
              tunnel: w245 -> [w250 w256 w262]
              frame "int32" {
                n76 = To Long Integer(number=w252) -> (32bit integer=w251:i32[][])
                n77 = call-poly "addArgument.vi"("argument list in"=w250, "data"=w251, "LabVIEW-Python-Interface in"=w255) -> ("argument list out"=w253:T5[], "LabVIEW-Python-Interface out"=w254:refnum<class "PyLVi.lvclass">)  [unwired: 6 in, 1 out]
              }
              frame "float64", Default {
                n78 = call-poly "addArgument.vi"("argument list in"=w256, "data"=w257, "LabVIEW-Python-Interface in"=w260) -> ("argument list out"=w258:T5[], "LabVIEW-Python-Interface out"=w259:refnum<class "PyLVi.lvclass">)  [unwired: 6 in, 1 out]
              }
              frame "complex128" {
                n79 = call-poly "addArgument.vi"("argument list in"=w262, "data"="multi:2darray send complex", "LabVIEW-Python-Interface in"=w265) -> ("argument list out"=w263:T5[], "LabVIEW-Python-Interface out"=w264:refnum<class "PyLVi.lvclass">)  [unwired: 6 in, 1 out]
              }
            }
          }
          frame "dict" {
            n80 = Flatten To JSON(enable LabVIEW extensions? (T)=FALSE, anything="multi:dict send") -> (JSON string=w266:string)  [unwired: 1 in, 1 out]
            n81 = call-poly "addArgument.vi"("argument list in"=w269, "JSON string"=w266, "LabVIEW-Python-Interface in"=w272) -> ("argument list out"=w270:T5[], "LabVIEW-Python-Interface out"=w271:refnum<class "PyLVi.lvclass">)  [unwired: 6 in, 1 out]
          }
        }
        n82 = local write "multi:argument send"(w185) -> ()
      }
      event "multi:clear last argument": Value Change {
        # "delete last element"
        n83 = event-data() -> ()  [unwired: 1 in, 6 out]
        n84 = local read "multi:argument send"() -> (w276:T5[])
        n85 = Array Size(array=w276) -> (size(s)=w274:i32)
        n86 = Decrement(x=w274) -> (x-1=w275:i32)
        n87 = Delete From Array(array=w276, length=1, index=w275) -> (array with subset deleted=w278:T5[])  [unwired: 1 out]
        n88 = local write "multi:argument send"(w278) -> ()
      }
      event "multi:call function": Value Change {
        n89 = event-data() -> ()  [unwired: 1 in, 6 out]
        n90 = local read "multi:argument send"() -> (w280:T5[])
        n91 = call "callFunction.vi"("object"="multi:object", "argument list in"=w280, "function"="multi:function", "LabVIEW-Python-Interface in"=w284) -> ("return list"=w279:T5[], "LabVIEW-Python-Interface out"=w283:refnum<class "PyLVi.lvclass">)  [unwired: 5 in, 1 out]
        n92 = local write "multi:argument receive"(w279) -> ()
      }
      event "multi:get return parameter": Value Change {
        n93 = event-data() -> ()  [unwired: 1 in, 6 out]
        n94 = local read "multi:argument receive"() -> (w286:T5[])
        n95 = local read "multi:data type"() -> (w288:T4)
        n96 = local read "multi:argtype"() -> (w287:T3)
        n97 = case shown="\"ndarray2d\"" w287 {
          tunnel: w290 -> [w295 w300 w306 w327 w348 w371]
          tunnel: [w294 w299 w305 w326 w347 w370] -> w289
          tunnel: w288 -> [_ _ w304 w325 w346 _]
          tunnel: w286 -> [w293 w296 w303 w324 w345 w365]
          tunnel: [w292 w297 w302 w323 w344 w364] -> w285
          frame "bool", Default {
            n98 = call-poly "getReturn.vi"("return list in"=w293, "LabVIEW-Python-Interface in"=w295) -> ("return list out"=w292:T5[], "data"=→"multi:bool receive":bool, "LabVIEW-Python-Interface out"=w294:refnum<class "PyLVi.lvclass">)  [unwired: 6 in, 1 out]
          }
          frame "string" {
            n99 = call-poly "getReturn.vi"("return list in"=w296, "LabVIEW-Python-Interface in"=w300) -> ("return list out"=w297:T5[], "data out"=→"multi:string receive":string, "LabVIEW-Python-Interface out"=w299:refnum<class "PyLVi.lvclass">)  [unwired: 6 in, 1 out]
          }
          frame "numeric" {
            n100 = case shown="\"complex128\"" w304 {
              tunnel: w306 -> [w311 w316 w321]
              tunnel: [w310 w315 w320] -> w305
              tunnel: [w309 w314 _] -> w301
              tunnel: w303 -> [w308 w313 w319]
              tunnel: [w307 w312 w318] -> w302
              frame "int32" {
                n101 = call-poly "getReturn.vi"("return list in"=w308, "LabVIEW-Python-Interface in"=w311) -> ("return list out"=w307:T5[], "data out"=w309:i32, "LabVIEW-Python-Interface out"=w310:refnum<class "PyLVi.lvclass">)  [unwired: 6 in, 1 out]
              }
              frame "float64", Default {
                n102 = call-poly "getReturn.vi"("return list in"=w313, "LabVIEW-Python-Interface in"=w316) -> ("return list out"=w312:T5[], "data out"=w314:dbl, "LabVIEW-Python-Interface out"=w315:refnum<class "PyLVi.lvclass">)  [unwired: 6 in, 1 out]
              }
              frame "complex128" {
                n103 = call-poly "getReturn.vi"("return list in"=w319, "LabVIEW-Python-Interface in"=w321) -> ("return list out"=w318:T5[], "data out"=→"multi:numeric receive complex":cdb, "LabVIEW-Python-Interface out"=w320:refnum<class "PyLVi.lvclass">)  [unwired: 6 in, 1 out]
              }
            }
            "multi:numeric receive" <- w301
          }
          frame "ndarray" {
            n104 = case shown="\"complex128\"" w325 {
              tunnel: w327 -> [w332 w337 w342]
              tunnel: [w331 w336 w341] -> w326
              tunnel: [w330 w335 _] -> w322
              tunnel: w324 -> [w329 w334 w340]
              tunnel: [w328 w333 w339] -> w323
              frame "int32" {
                n105 = call-poly "getReturn.vi"("return list in"=w329, "LabVIEW-Python-Interface in"=w332) -> ("return list out"=w328:T5[], "data out"=w330:i32[], "LabVIEW-Python-Interface out"=w331:refnum<class "PyLVi.lvclass">)  [unwired: 6 in, 1 out]
              }
              frame "float64", Default {
                n106 = call-poly "getReturn.vi"("return list in"=w334, "LabVIEW-Python-Interface in"=w337) -> ("return list out"=w333:T5[], "data out"=w335:dbl[], "LabVIEW-Python-Interface out"=w336:refnum<class "PyLVi.lvclass">)  [unwired: 6 in, 1 out]
              }
              frame "complex128" {
                n107 = call-poly "getReturn.vi"("return list in"=w340, "LabVIEW-Python-Interface in"=w342) -> ("return list out"=w339:T5[], "data out"=→"multi:array receive complex":cdb[], "LabVIEW-Python-Interface out"=w341:refnum<class "PyLVi.lvclass">)  [unwired: 6 in, 1 out]
              }
            }
            "multi:array receive" <- w322
          }
          frame "ndarray2d" {
            n108 = case shown="\"complex128\"" w346 {
              tunnel: w348 -> [w353 w358 w363]
              tunnel: [w352 w357 w362] -> w347
              tunnel: [w351 w356 _] -> w343
              tunnel: w345 -> [w350 w355 w361]
              tunnel: [w349 w354 w360] -> w344
              frame "int32" {
                n109 = call-poly "getReturn.vi"("return list in"=w350, "LabVIEW-Python-Interface in"=w353) -> ("return list out"=w349:T5[], "data out"=w351:i32[][], "LabVIEW-Python-Interface out"=w352:refnum<class "PyLVi.lvclass">)  [unwired: 6 in, 1 out]
              }
              frame "float64", Default {
                n110 = call-poly "getReturn.vi"("return list in"=w355, "LabVIEW-Python-Interface in"=w358) -> ("return list out"=w354:T5[], "data out"=w356:dbl[][], "LabVIEW-Python-Interface out"=w357:refnum<class "PyLVi.lvclass">)  [unwired: 6 in, 1 out]
              }
              frame "complex128" {
                n111 = call-poly "getReturn.vi"("return list in"=w361, "LabVIEW-Python-Interface in"=w363) -> ("return list out"=w360:T5[], "data out"=→"multi:2darray receive complex":cdb[][], "LabVIEW-Python-Interface out"=w362:refnum<class "PyLVi.lvclass">)  [unwired: 6 in, 1 out]
              }
            }
            "multi:2darray receive" <- w343
          }
          frame "dict" {
            n112 = call-poly "getReturn.vi"("return list in"=w365, "LabVIEW-Python-Interface in"=w371) -> ("return list out"=w364:T5[], "data out"=w368:string, "LabVIEW-Python-Interface out"=w370:refnum<class "PyLVi.lvclass">)  [unwired: 6 in, 1 out]
            n113 = Unflatten From JSON(enable LabVIEW extensions? (T)=TRUE, JSON string=w368, type and defaults=T2 {"Name"="tcp://127.0.0.1:5555", "Number"=0.0, "Boolean"=FALSE, "Array"=[2.0, 2.0, 4.0, 4.0]} ("single:dict receive")) -> (value=→"multi:dict receive":T2)  [unwired: 4 in, 1 out]
          }
        }
        n114 = local write "multi:argument receive"(w285) -> ()
      }
      event "close connection": Value Change {
        n115 = event-data() -> ()  [unwired: 1 in, 6 out]
        n116 = call "closeConnection.vi"("LabVIEW-Python-Interface in"=w373) -> ("LabVIEW-Python-Interface out"=w372:refnum<class "PyLVi.lvclass">)  [unwired: 9 in, 1 out]
      }
      event "prop:set": Value Change {
        n117 = event-data() -> ()  [unwired: 1 in, 6 out]
        n118 = case shown="\"ndarray\"" "prop:argtype" {
          tunnel: w378 -> [w384 w389 w395 w417 w439 w462]
          tunnel: "prop:object" -> [w382 w387 w394 w416 w438 w460]
          tunnel: "prop:property" -> [w381 w386 w393 w415 w437 w459]
          tunnel: "prop:data type" -> [_ _ w392 w414 w436 _]
          tunnel: [w383 w388 w390 w413 w435 w461] -> w374
          frame "bool", Default {
            n119 = call-poly "setAttribute.vi"("object"=w382, "data"="prop:bool set", "attribute"=w381, "LabVIEW-Python-Interface in"=w384) -> ("LabVIEW-Python-Interface out"=w383:refnum<class "PyLVi.lvclass">)  [unwired: 6 in, 1 out]
          }
          frame "string" {
            n120 = call-poly "setAttribute.vi"("object"=w387, "data"="prop:string set", "attribute"=w386, "LabVIEW-Python-Interface in"=w389) -> ("LabVIEW-Python-Interface out"=w388:refnum<class "PyLVi.lvclass">)  [unwired: 6 in, 1 out]
          }
          frame "numeric" {
            n121 = case shown="\"complex128\"" w392 {
              tunnel: w395 -> [w401 w406 w411]
              tunnel: w394 -> [w400 w405 w410]
              tunnel: w393 -> [w399 w404 w409]
              tunnel: "prop:numeric set" -> [w396 w402 _]
              tunnel: [w397 w403 w408] -> w390
              frame "int32" {
                n122 = To Long Integer(number=w396) -> (32bit integer=w398:i32)
                n123 = call-poly "setAttribute.vi"("object"=w400, "data"=w398, "attribute"=w399, "LabVIEW-Python-Interface in"=w401) -> ("LabVIEW-Python-Interface out"=w397:refnum<class "PyLVi.lvclass">)  [unwired: 6 in, 1 out]
              }
              frame "float64", Default {
                n124 = call-poly "setAttribute.vi"("object"=w405, "data"=w402, "attribute"=w404, "LabVIEW-Python-Interface in"=w406) -> ("LabVIEW-Python-Interface out"=w403:refnum<class "PyLVi.lvclass">)  [unwired: 6 in, 1 out]
              }
              frame "complex128" {
                n125 = call-poly "setAttribute.vi"("object"=w410, "data"="prop:numeric set complex", "attribute"=w409, "LabVIEW-Python-Interface in"=w411) -> ("LabVIEW-Python-Interface out"=w408:refnum<class "PyLVi.lvclass">)  [unwired: 6 in, 1 out]
              }
            }
          }
          frame "ndarray" {
            n126 = case shown="\"complex128\"" w414 {
              tunnel: w417 -> [w423 w428 w433]
              tunnel: w416 -> [w422 w427 w432]
              tunnel: w415 -> [w421 w426 w431]
              tunnel: "prop:array set" -> [w419 w424 _]
              tunnel: [w418 w425 w430] -> w413
              frame "int32" {
                n127 = To Long Integer(number=w419) -> (32bit integer=w420:i32[])
                n128 = call-poly "setAttribute.vi"("object"=w422, "data"=w420, "attribute"=w421, "LabVIEW-Python-Interface in"=w423) -> ("LabVIEW-Python-Interface out"=w418:refnum<class "PyLVi.lvclass">)  [unwired: 6 in, 1 out]
              }
              frame "float64", Default {
                n129 = call-poly "setAttribute.vi"("object"=w427, "data"=w424, "attribute"=w426, "LabVIEW-Python-Interface in"=w428) -> ("LabVIEW-Python-Interface out"=w425:refnum<class "PyLVi.lvclass">)  [unwired: 6 in, 1 out]
              }
              frame "complex128" {
                n130 = call-poly "setAttribute.vi"("object"=w432, "data"="prop:array set complex", "attribute"=w431, "LabVIEW-Python-Interface in"=w433) -> ("LabVIEW-Python-Interface out"=w430:refnum<class "PyLVi.lvclass">)  [unwired: 6 in, 1 out]
              }
            }
          }
          frame "ndarray2d" {
            n131 = case shown="\"complex128\"" w436 {
              tunnel: w439 -> [w445 w450 w455]
              tunnel: w438 -> [w444 w449 w454]
              tunnel: w437 -> [w443 w448 w453]
              tunnel: "prop:2darray set" -> [w441 w446 _]
              tunnel: [w440 w447 w452] -> w435
              frame "int32" {
                n132 = To Long Integer(number=w441) -> (32bit integer=w442:i32[][])
                n133 = call-poly "setAttribute.vi"("object"=w444, "data"=w442, "attribute"=w443, "LabVIEW-Python-Interface in"=w445) -> ("LabVIEW-Python-Interface out"=w440:refnum<class "PyLVi.lvclass">)  [unwired: 6 in, 1 out]
              }
              frame "float64", Default {
                n134 = call-poly "setAttribute.vi"("object"=w449, "data"=w446, "attribute"=w448, "LabVIEW-Python-Interface in"=w450) -> ("LabVIEW-Python-Interface out"=w447:refnum<class "PyLVi.lvclass">)  [unwired: 6 in, 1 out]
              }
              frame "complex128" {
                n135 = call-poly "setAttribute.vi"("object"=w454, "data"="prop:2darray set complex", "attribute"=w453, "LabVIEW-Python-Interface in"=w455) -> ("LabVIEW-Python-Interface out"=w452:refnum<class "PyLVi.lvclass">)  [unwired: 6 in, 1 out]
              }
            }
          }
          frame "dict" {
            n136 = Flatten To JSON(enable LabVIEW extensions? (T)=FALSE, anything="prop:dict set") -> (JSON string=w457:string)  [unwired: 1 in, 1 out]
            n137 = call-poly "setAttribute.vi"("object"=w460, "data dict"=w457, "attribute"=w459, "LabVIEW-Python-Interface in"=w462) -> ("LabVIEW-Python-Interface out"=w461:refnum<class "PyLVi.lvclass">)  [unwired: 6 in, 1 out]
          }
        }
      }
      event "prop:get": Value Change {
        n138 = event-data() -> ()  [unwired: 1 in, 6 out]
        n139 = local read "prop:data type"() -> (w463:T4)
        n140 = local read "prop:property"() -> (w465:string)
        n141 = local read "prop:argtype"() -> (w464:T3)
        n142 = local read "prop:object"() -> (w466:string)
        n143 = case shown="\"numeric\"" w464 {
          tunnel: w468 -> [w473 w478 w484 w505 w526 w549]
          tunnel: [w472 w477 w483 w504 w525 w548] -> w467
          tunnel: w466 -> [w471 w476 w482 w503 w524 w547]
          tunnel: w465 -> [w470 w475 w481 w502 w523 w546]
          tunnel: w463 -> [_ _ w480 w501 w522 _]
          frame "bool", Default {
            n144 = call-poly "getAttribute.vi"("object"=w471, "attribute"=w470, "LabVIEW-Python-Interface in"=w473) -> ("data"=→"prop:bool get":bool, "LabVIEW-Python-Interface out"=w472:refnum<class "PyLVi.lvclass">)  [unwired: 6 in, 1 out]
          }
          frame "string" {
            n145 = call-poly "getAttribute.vi"("object"=w476, "attribute"=w475, "LabVIEW-Python-Interface in"=w478) -> ("data"=→"grop:string get":string, "LabVIEW-Python-Interface out"=w477:refnum<class "PyLVi.lvclass">)  [unwired: 6 in, 1 out]
          }
          frame "numeric" {
            n146 = case shown="\"complex128\"" w480 {
              tunnel: w484 -> [w489 w494 w499]
              tunnel: [w488 w493 w498] -> w483
              tunnel: w482 -> [w487 w492 w497]
              tunnel: w481 -> [w486 w491 w496]
              tunnel: [w485 w490 _] -> w479
              frame "int32" {
                n147 = call-poly "getAttribute.vi"("object"=w487, "attribute"=w486, "LabVIEW-Python-Interface in"=w489) -> ("data"=w485:i32, "LabVIEW-Python-Interface out"=w488:refnum<class "PyLVi.lvclass">)  [unwired: 6 in, 1 out]
              }
              frame "float64", Default {
                n148 = call-poly "getAttribute.vi"("object"=w492, "attribute"=w491, "LabVIEW-Python-Interface in"=w494) -> ("data"=w490:dbl, "LabVIEW-Python-Interface out"=w493:refnum<class "PyLVi.lvclass">)  [unwired: 6 in, 1 out]
              }
              frame "complex128" {
                n149 = call-poly "getAttribute.vi"("object"=w497, "attribute"=w496, "LabVIEW-Python-Interface in"=w499) -> ("data"=→"prop:numeric get complex":cdb, "LabVIEW-Python-Interface out"=w498:refnum<class "PyLVi.lvclass">)  [unwired: 6 in, 1 out]
              }
            }
            "prop:numeric get" <- w479
          }
          frame "ndarray" {
            n150 = case shown="\"complex128\"" w501 {
              tunnel: w505 -> [w510 w515 w520]
              tunnel: [w509 w514 w519] -> w504
              tunnel: w503 -> [w508 w513 w518]
              tunnel: w502 -> [w507 w512 w517]
              tunnel: [w506 w511 _] -> w500
              frame "int32" {
                n151 = call-poly "getAttribute.vi"("object"=w508, "attribute"=w507, "LabVIEW-Python-Interface in"=w510) -> ("data"=w506:i32[], "LabVIEW-Python-Interface out"=w509:refnum<class "PyLVi.lvclass">)  [unwired: 6 in, 1 out]
              }
              frame "float64", Default {
                n152 = call-poly "getAttribute.vi"("object"=w513, "attribute"=w512, "LabVIEW-Python-Interface in"=w515) -> ("data"=w511:dbl[], "LabVIEW-Python-Interface out"=w514:refnum<class "PyLVi.lvclass">)  [unwired: 6 in, 1 out]
              }
              frame "complex128" {
                n153 = call-poly "getAttribute.vi"("object"=w518, "attribute"=w517, "LabVIEW-Python-Interface in"=w520) -> ("data"=→"prop:array get complex":cdb[], "LabVIEW-Python-Interface out"=w519:refnum<class "PyLVi.lvclass">)  [unwired: 6 in, 1 out]
              }
            }
            "prop:array get" <- w500
          }
          frame "ndarray2d" {
            n154 = case shown="\"complex128\"" w522 {
              tunnel: w526 -> [w531 w536 w541]
              tunnel: [w530 w535 w540] -> w525
              tunnel: w524 -> [w529 w534 w539]
              tunnel: w523 -> [w528 w533 w538]
              tunnel: [w527 w532 _] -> w521
              frame "int32" {
                n155 = call-poly "getAttribute.vi"("object"=w529, "attribute"=w528, "LabVIEW-Python-Interface in"=w531) -> ("data"=w527:i32[][], "LabVIEW-Python-Interface out"=w530:refnum<class "PyLVi.lvclass">)  [unwired: 6 in, 1 out]
              }
              frame "float64", Default {
                n156 = call-poly "getAttribute.vi"("object"=w534, "attribute"=w533, "LabVIEW-Python-Interface in"=w536) -> ("data"=w532:dbl[][], "LabVIEW-Python-Interface out"=w535:refnum<class "PyLVi.lvclass">)  [unwired: 6 in, 1 out]
              }
              frame "complex128" {
                n157 = call-poly "getAttribute.vi"("object"=w539, "attribute"=w538, "LabVIEW-Python-Interface in"=w541) -> ("data"=→"prop:2darray receive complex":cdb[][], "LabVIEW-Python-Interface out"=w540:refnum<class "PyLVi.lvclass">)  [unwired: 6 in, 1 out]
              }
            }
            "prop:2darray get" <- w521
          }
          frame "dict" {
            n158 = call-poly "getAttribute.vi"("object"=w547, "attribute"=w546, "LabVIEW-Python-Interface in"=w549) -> ("data"=w544:string, "LabVIEW-Python-Interface out"=w548:refnum<class "PyLVi.lvclass">)  [unwired: 6 in, 1 out]
            n159 = Unflatten From JSON(enable LabVIEW extensions? (T)=TRUE, JSON string=w544, type and defaults=T2 {"Name"="tcp://127.0.0.1:5555", "Number"=0.0, "Boolean"=FALSE, "Array"=[2.0, 2.0, 4.0, 4.0]} ("single:dict receive")) -> (value=→"prop:dict get":T2)  [unwired: 4 in, 1 out]
          }
        }
      }
    }
  }
  n160 = local write "Tab Control"(T1."Connection" ("Tab Control")) -> ()
  "multi:argument send" <- w2
  "multi:argument receive" <- w2
